vi "define columns.vi"(10 "enum references":refnum<vi>[](array[refnum])) -> (2 "Column Definition":T1[](array[typedef]) {"MinWidth" min=2 step=1; "AutoSizeMode" items=["None"=1, "ColumnHeader"=2, "AllCellsExceptHeader"=4, "AllCells"=6, "DisplayedCellsExceptHeader"=8, "DisplayedCells"=10, "Fill"=16]; "FillWeight" min=1 max=100})   [LabVIEW 2013, in "Shared Memory Editor Node.lvclass"]
doc: "Copyright 2016 National Instruments Corporation\n\nLicensed under the Apache License, Version 2.0 (the \"License\"); you may not use this file except in compliance with the License. You may obtain a copy of the License at http://www.apache.org/licenses/LICENSE-2.0\nUnless required by applicable law or agreed to in writing, software distributed under the License is distributed on an \"AS IS\" BASIS, WITHOUT WARRANTIES OR CONDITIONS OF ANY KIND, either express or implied. See the License for the specific language governing permissions and limitations under the License."
uses:
  Shared Memory Editor Node.lvclass
  <vilib>/NI/DCAF Table API/Column/Column Descriptor.ctl
  <vilib>/NI/DCAF Table API/Column/Column Type.ctl
  <vilib>/NI/Tag Bus/tag/Data Type.ctl
  <vilib>/NI/DCAF Table API/Table Manager/Call Back Ref Type Def.ctl
  <vilib>/NI/DCAF/Tag Editor Core/Configuration Editor/Classes/Engine Parent/Engine Parent Editor Node.lvclass
  <vilib>/NI/DCAF/Tag Editor Core/Configuration Editor/Classes/Module editor node/module editor node.lvclass
  <vilib>/NI/DCAF Table API/Column/Column.lvclass
  <vilib>/NI/Tag Bus/tag/tag descriptor.lvclass
  <vilib>/NI/DCAF Table API/Table Manager/Table Manager.lvclass
  <vilib>/NI/DCAF Table API/Mapping Column/Mapping Column.lvclass
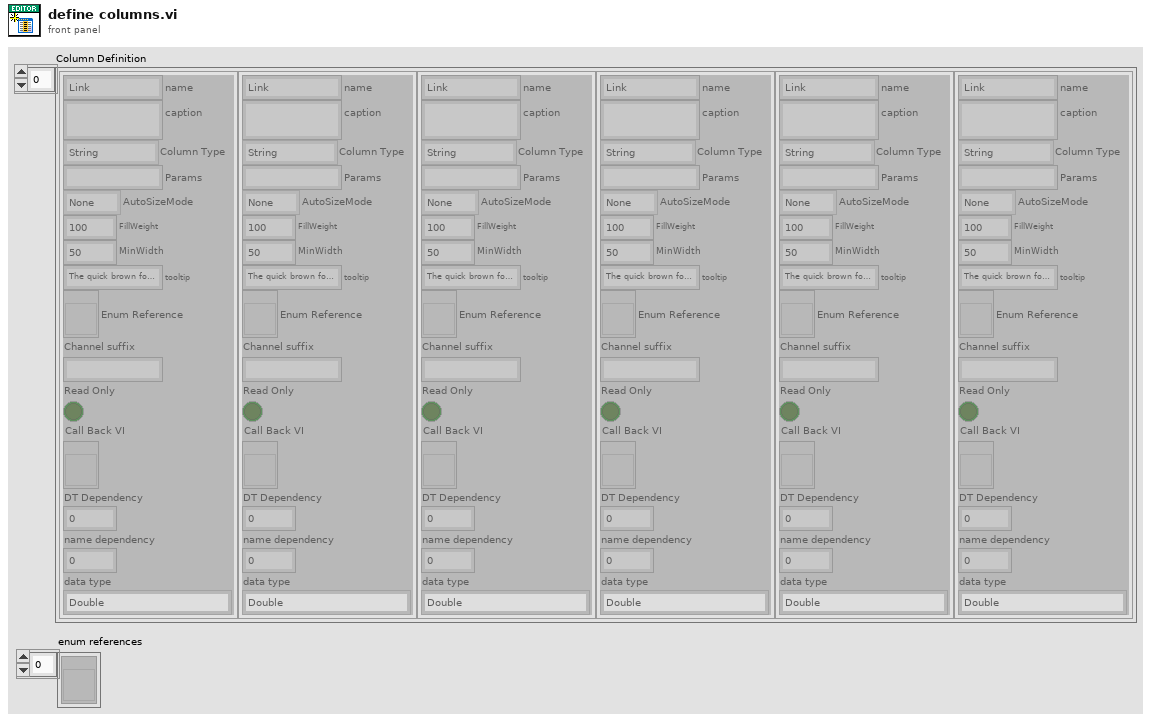
[diagram p1: front panel]
types:
  T1 = typedef "Table Manager.lvlib/Column.lvclass/Column Descriptor.ctl" = cluster{"name":string, "caption":string, "Column Type":T2, "Params":string, "AutoSizeMode":i32, "FillWeight":sgl, "MinWidth":u32, "tooltip":string, "Enum Reference":refnum<vi>, "Channel suffix":string, "Read Only":bool, "Call Back VI":T3, "DT Dependency":i32, "name dependency":i32, "data type":T4}
  T2 = typedef "Table Manager.lvlib/Column.lvclass/Column Type.ctl" = enum16{"String", "Mapping", "Channel Name", "Tag", "Enum", "Data Type", "Numeric"}
  T3 = typedef "Table Manager.lvlib/Table Manager.lvclass/Call Back Ref Type Def.ctl" = refnum<vi>
  T4 = typedef "tag bus.lvlib/tag descriptor.lvclass/Data Type.ctl" = enum16{"Double", "Single", "I64", "I32", "I16", "I8", "U64", "U32", "U16", "U8", "Boolean", "String", "Array of Double", "Array of Single", "Array of I64", "Array of I32", "Array of I16", "Array of I8", "Array of U64", "Array of U32", "Array of U16", "Array of U8", "Array of Boolean", "Array of String"}
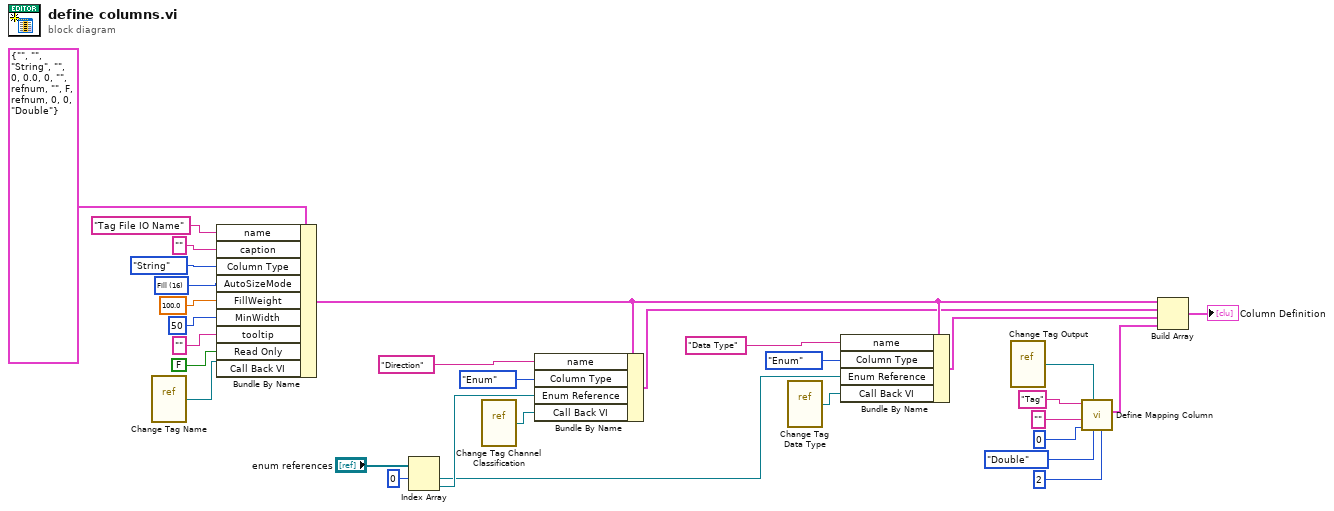
[diagram p0: block diagram]
diagram:
  w22 = 16 items=["None"=1, "ColumnHeader"=2, "AllCellsExceptHeader"=4, "AllCells"=6, "DisplayedCellsExceptHeader"=8, "DisplayedCells"=10, "Fill"=16] ("AutoSizeMode")
  n1 = vi-ref "Change Tag Name.vi"() -> (w18:refnum<vi>)
  n2 = Bundle By Name(cluster=T1 {"name"="", "caption"="", "Column Type"=enum."String", "Params"="", "AutoSizeMode"=0, "FillWeight"=0.0, "MinWidth"=0, "tooltip"="", "Enum Reference"=refnum, "Channel suffix"="", "Read Only"=FALSE, "Call Back VI"=refnum, "DT Dependency"=0, "name dependency"=0, "data type"=enum."Double"} ("Table Manager.lvlib:Column.lvclass:Column Descriptor"), "name"="Tag File IO Name", "caption"="", "Column Type"=Column_Type."String", "AutoSizeMode"=w22, "FillWeight"=sgl 100.0, "MinWidth"=u32 50, "tooltip"="", "Read Only"=FALSE, "Call Back VI"=w18) -> (w7:T1)
  n3 = Index Array(array="enum references", index #1=0 ("index")) -> (element #1=w2:refnum<vi>, element #2=w3:refnum<vi>)  [unwired: 1 in]
  n4 = vi-ref "Change Tag Channel Classification.vi"() -> (w12:refnum<vi>)
  n5 = Bundle By Name(cluster=w7, "name"="Direction", "Column Type"=Column_Type."Enum", "Enum Reference"=w3, "Call Back VI"=w12) -> (w6:T1)
  n6 = vi-ref "Change Tag Data Type.vi"() -> (w19:refnum<vi>)
  n7 = Bundle By Name(cluster=w7, "name"="Data Type", "Column Type"=Column_Type."Enum", "Enum Reference"=w2, "Call Back VI"=w19) -> (w8:T1)
  n8 = vi-ref "Change Tag Output.vi"() -> (w17:refnum<vi>)
  n9 = call <vilib>:"Define Mapping Column.vi"("DT Dependency"=2, "data type"=Data_Type."Double", "Call Back VI"=w17, "name dependency"=0, "Channel suffix"="", "name"="Tag") -> ("Table Manager.lvlib:Column.lvclass:Column Descriptor"=w9:T1)  [unwired: 5 in]
  n10 = Build Array(w7, w6, w8, w9) -> (→"Column Definition":T1[])
